vi "LookUpBand.vi"(8 "error in (no error)":errorcluster, 10 "MetricDefinitionInstanceId":string, 11 "Metric Cache":variant) -> (0 "error out":errorcluster, 2 "SpectralBand":T1, 3 "Metric Cache Out":variant)   [LabVIEW 2017, in "AnalysisHelper.lvlib"]
uses:
  <vilib>/addons/InsightCM/Utilities/Analysis/Shared/AnalysisHelper.lvlib
  <vilib>/addons/InsightCM/Utilities/Analysis/Shared/controls/BandConfig.ctl
  <vilib>/addons/InsightCM/Utilities/Analysis/Shared/controls/BandDomain.ctl
  <vilib>/addons/InsightCM/Utilities/Analysis/Shared/controls/BandCalculation.ctl
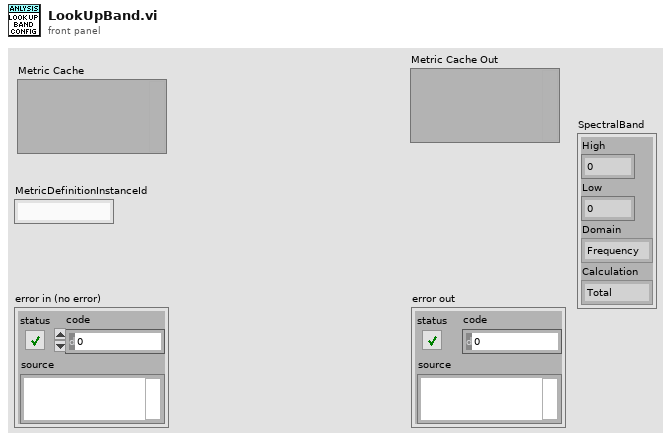
[diagram p1: front panel]
types:
  T1 = typedef "AnalysisHelper.lvlib/BandConfig.ctl" = cluster{"High":dbl, "Low":dbl, "Domain":T2, "Calculation":T3}
  T2 = typedef "AnalysisHelper.lvlib/BandDomain.ctl" = enum16{"Frequency", "CPM", "Orders"}
  T3 = typedef "AnalysisHelper.lvlib/BandCalculation.ctl" = enum16{"Total", "Max", "Phase"}
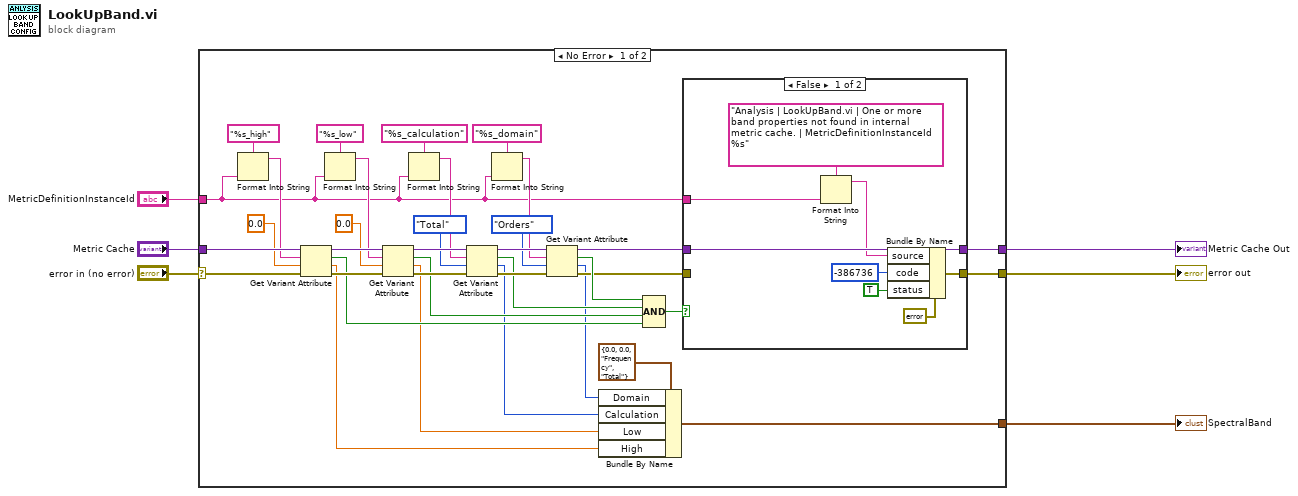
[diagram p0: block diagram]
diagram:
  n1 = case shown="No Error" "error in (no error)" {
    selector: "error in (no error)" -> [w27 w53]
    tunnel: "Metric Cache" -> [w32 w54]
    tunnel: "MetricDefinitionInstanceId" -> [w19 _]
    tunnel: [w20 w53] -> w4
    tunnel: [w18 w54] -> w3
    tunnel: [w9 _] -> w1
    frame No Error {
      n2 = Format Into String(format string="%s_high", w19) -> (resulting string=w31:string)  [unwired: 2 in, 1 out]
      n3 = Get Variant Attribute(Variant=w32, name=w31, default value (empty Variant)=sgl 0.0 ("default (0 DBL)"), error in=w27) -> (duplicate Variant=w33:variant, found=w23:bool, value=w10:sgl, error out=w38:errorcluster)
      n4 = Format Into String(format string="%s_low", w19) -> (resulting string=w30:string)  [unwired: 2 in, 1 out]
      n5 = Get Variant Attribute(Variant=w33, name=w30, default value (empty Variant)=sgl 0.0 ("default (0 DBL)"), error in=w38) -> (duplicate Variant=w34:variant, found=w24:bool, value=w11:sgl, error out=w37:errorcluster)
      n6 = Format Into String(format string="%s_calculation", w19) -> (resulting string=w29:string)  [unwired: 2 in, 1 out]
      n7 = Get Variant Attribute(Variant=w34, name=w29, default value (empty Variant)=BandCalculation."Total" ("Spectral Band Calculation"), error in=w37) -> (duplicate Variant=w35:variant, found=w25:bool, value=w12:T3, error out=w36:errorcluster)
      n8 = Format Into String(format string="%s_domain", w19) -> (resulting string=w28:string)  [unwired: 2 in, 1 out]
      n9 = Get Variant Attribute(Variant=w35, name=w28, default value (empty Variant)=BandDomain."Orders" ("Spectral Band Domain"), error in=w36) -> (duplicate Variant=w17:variant, found=w26:bool, value=w13:T2, error out=w21:errorcluster)
      n10 = Bundle By Name(cluster=T1 {"High"=0.0, "Low"=0.0, "Domain"=enum."Frequency", "Calculation"=enum."Total"} ("SpectralBand"), "Domain"=w13, "Calculation"=w12, "Low"=w11, "High"=w10) -> (w9:T1)
      n11 = Compound Arithmetic op=AND(w26, w25, w24, w23) -> (w22:bool)
      n12 = case shown="False" w22 {
        tunnel: w21 -> [_ w52]
        tunnel: [w50 w52] -> w20
        tunnel: w19 -> [w48 _]
        tunnel: [w46 w51] -> w18
        tunnel: w17 -> [w46 w51]
        frame False {
          n13 = Format Into String(format string="Analysis | LookUpBand.vi | One or more band properties not found in internal metric cache. | MetricDefinitionInstanceId %s" ("source"), w48) -> (resulting string=w45:string)  [unwired: 2 in, 1 out]
          n14 = Bundle By Name(cluster=errorcluster {"status"=FALSE, "code"=0, "source"=""} ("error out"), "source"=w45, "code"=-386736, "status"=TRUE) -> (w50:errorcluster)
        }
        frame True {
        }
      }
    }
    frame Error {
    }
  }
  "error out" <- w4
  "Metric Cache Out" <- w3
  "SpectralBand" <- w1
